vi "Write sp.vi"(8 "error in (no error)":errorcluster, 10 "sp":dbl, 11 "Update Device Setpoint MSG in":refnum<class "Update Device Setpoint MSG.lvclass">) -> (0 "error out":errorcluster, 3 "Update Device Setpoint MSG out":refnum<class "Update Device Setpoint MSG.lvclass">)   [LabVIEW 2017, in "Update Device Setpoint MSG.lvclass"]
uses:
  Update Device Setpoint MSG.lvclass
  Update Device Setpoint MSG.lvclass/Update Device Setpoint MSG.ctl
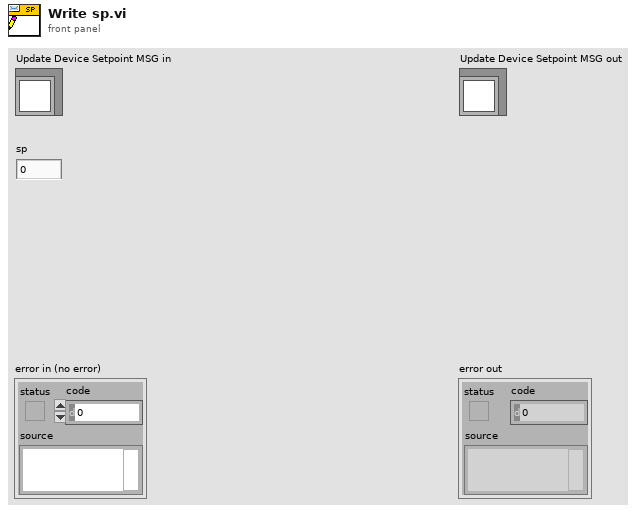
[diagram p1: front panel]
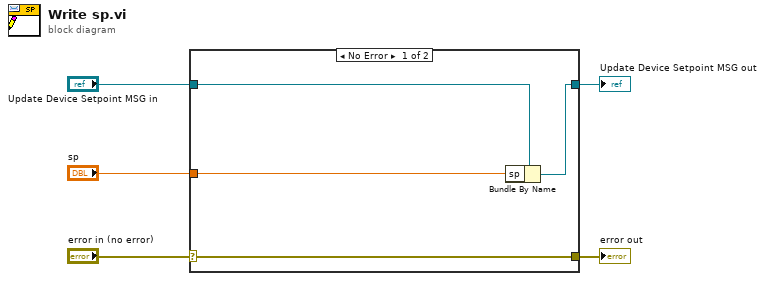
[diagram p0: block diagram]
diagram:
  n1 = case shown="No Error" "error in (no error)" {
    selector: "error in (no error)" -> [w9 w10]
    tunnel: [w9 w10] -> w4
    tunnel: [w7 w11] -> w2
    tunnel: "Update Device Setpoint MSG in" -> [w8 w11]
    tunnel: "sp" -> [w6 _]
    frame No Error {
      n2 = Bundle By Name(cluster=w8, "sp"=w6) -> (w7:refnum<class "Update Device Setpoint MSG.lvclass">)
    }
    frame Error {
    }
  }
  "error out" <- w4
  "Update Device Setpoint MSG out" <- w2
